vi "Add notifier.vi"(8 "error in (no error)":errorcluster, 10 "notifier":refnum<notifier>, 11 "DAQmxTaksContainer_General in":refnum<class "DAQmxTaksContainer_General.lvclass">) -> (0 "error out":errorcluster, 3 "DAQmxTaksContainer_General out":refnum<class "DAQmxTaksContainer_General.lvclass">)   [LabVIEW 2015, in "DAQmxTaksContainer_General.lvclass"]
uses:
  DAQmxTaksContainer_General.lvclass
  DAQmxTaksContainer_General.lvclass/DAQmxTaksContainer_General.ctl
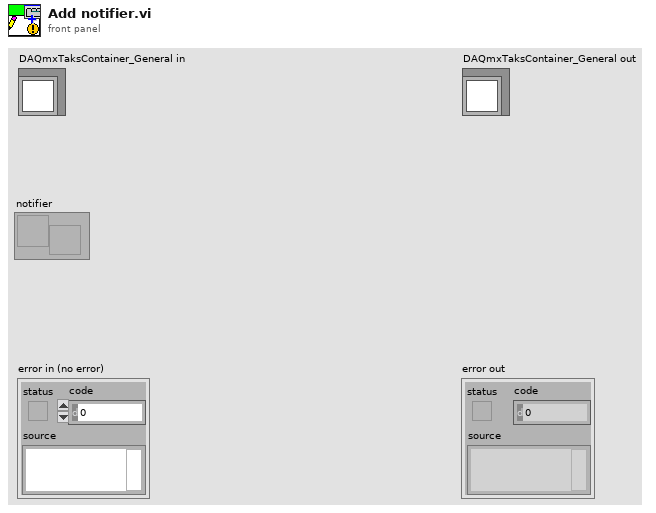
[diagram p1: front panel]
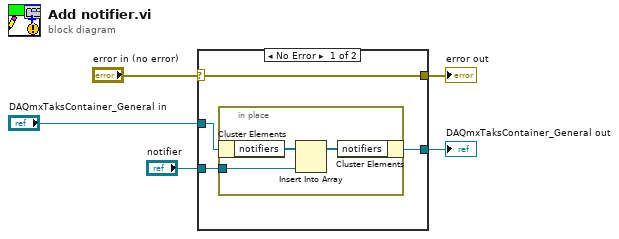
[diagram p0: block diagram]
diagram:
  n1 = case shown="No Error" "error in (no error)" {
    selector: "error in (no error)" -> [w9 w13]
    tunnel: [w9 w13] -> w4
    tunnel: [w7 w14] -> w2
    tunnel: "DAQmxTaksContainer_General in" -> [w8 w14]
    tunnel: "notifier" -> [w6 _]
    frame No Error {
      n2 = in-place {
        in-place-border: w6 -> [w10]
        n3 = in-place-cluster #1(w8) -> ("notifiers"=w12:refnum<notifier>[])
        n4 = Insert Into Array(array=w12, new element=w10) -> (w11:refnum<notifier>[])  [unwired: 1 in]
        n5 = in-place-cluster #1("notifiers"=w11) -> (w7:refnum<class "DAQmxTaksContainer_General.lvclass">)
      }
    }
    frame Error {
    }
  }
  "error out" <- w4
  "DAQmxTaksContainer_General out" <- w2
